vi "CSM Execute - Upgrade Debug Log History Method.vi"(6 "Mouse Position":T1, 8 "User VI Ref":refnum<vi>, 9 "Menu Item Tag Suffix":string, 10 "Remaining Items":refnum<vi>[](array[refnum]), 11 "Affected Items":T2) -> (0 "Fail transaction?":bool)   [LabVIEW 2017]
doc: "This VI is part of a plug-in for modifying the LabVIEW shortcut menus. This is the execute VI which is called when the shortcut menu is chosen by the user. It performs the action of the selected menu item."
uses:
  CSM Execute - Shortcut Menu Plug-In.ctl
  <vilib>/Utility/miscctls.llb/LVPositionTypeDef.ctl
  _csmHelper/API/Destroy.vi
  _csmHelper/usecase/Replace Debug Log History Method.vi
  _csmHelper/API/Create From Basic Refs.vi
  _csmHelper/CSM-Helper.lvclass
  _csmHelper/Utility/CSM-Helper Utility.lvlib
panel:
  # "All controls on this panel except \"Affected Items\" have been locked to prevent accidental edits. Changing the control names or types, other than the elements of the \"Affected Items\" cluster will make the VI unusable as a menu plugin.\n\nSee Context Help for each control for details about its use."
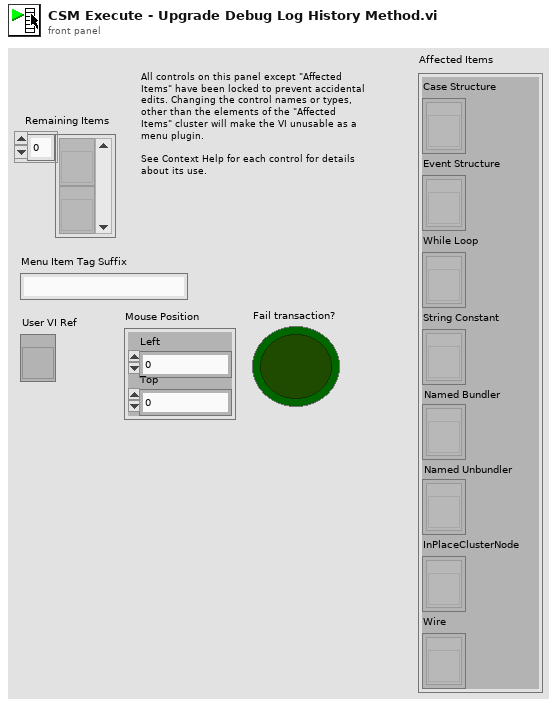
[diagram p1: front panel]
types:
  T1 = typedef "LVPositionTypeDef.ctl" = cluster{"Left":i32, "Top":i32}
  T2 = typedef "CSM Execute - Shortcut Menu Plug-In.ctl" = cluster{"Case Structure":refnum<vi>[], "Event Structure":refnum<vi>[], "While Loop":refnum<vi>[], "String Constant":refnum<vi>[], "Named Bundler":refnum<vi>[], "Named Unbundler":refnum<vi>[], "InPlaceClusterNode":refnum<vi>[], "Wire":refnum<vi>[]}
  T3 = typedef "CSM-Helper Utility.lvlib/CSM Basic Refs.ctl" = cluster{"VI":refnum<vi>, "While Loop":refnum<vi>, "Case Structure":refnum<vi>, "Parse State Queue":refnum<vi>, "Event Structure":refnum<vi>, "Type":T4, "InLvlibp":bool}
  T4 = typedef "CSM-Helper Utility.lvlib/CSM Module Type.ctl" = enum16{"Not a CSM", "JKISM", "CSM"}
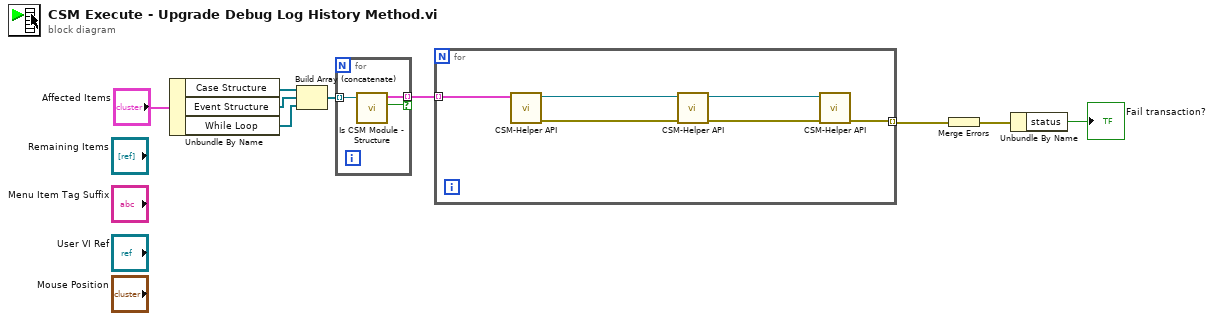
[diagram p0: block diagram]
diagram:
  n1 = Unbundle By Name("Affected Items") -> ("Case Structure"=w6:refnum<vi>[], "Event Structure"=w5:refnum<vi>[], "While Loop"=w4:refnum<vi>[])
  n2 = Build Array (concatenate)(w6, w5, w4) -> (w3:refnum<vi>[])
  n3 = for {
    tunnel: w3 -> [w12] mode=indexing
    tunnel: [w11] -> w1 mode=indexing if=w10
    n4 = call "Is CSM Module - Structure.vi"("Structure"=w12) -> ("Is CSM Module?"=w10:bool, "CSM Basic Refs"=w11:T3)  [unwired: 8 in, 1 out]
  }
  n5 = for {
    tunnel: [w14] -> w7 mode=indexing
    tunnel: w1 -> [w13] mode=indexing
    n6 = call-poly "CSM-Helper API.vi"("CSM Basic Refs"=w13) -> ("error out"=w15:errorcluster, "CSM-Helper.lvclass"=w18:refnum<class "CSM-Helper.lvclass">)  [unwired: 9 in]
    n7 = call-poly "CSM-Helper API.vi"("error in (no error)"=w15, "CSM-Helper in"=w18) -> ("error out"=w16:errorcluster, "CSM-Helper out"=w17:refnum<class "CSM-Helper.lvclass">)  [unwired: 8 in]
    n8 = call-poly "CSM-Helper API.vi"("error in (no error)"=w16, "CSM-Helper in"=w17) -> ("error out"=w14:errorcluster)  [unwired: 8 in, 1 out]
  }
  n9 = Merge Errors(w7) -> (w8:errorcluster)
  n10 = Unbundle By Name(w8) -> ("status"=→"Fail transaction?":bool)
